vi "ReadABLEConfiguration.vi"(8 "Error In":errorcluster, 11 "VI Path":path) -> (0 "Error Out":errorcluster, 3 "ABLE Configuration":T1)   [LabVIEW 2012]
uses:
  ABLEConfiguration.ctl
  DisplayConfiguration.ctl
  FolderConfiguration.ctl
  AlarmsConfiguration.ctl
  Keithley6485Configuration.ctl
  Keithley6482Configuration.ctl
  <vilib>/Utility/config.llb/Read Key (Boolean).vi
  <vilib>/Utility/config.llb/NI_LVConfig.lvlib
  libs/LV-Utilities/LV-Utilities.lvlib
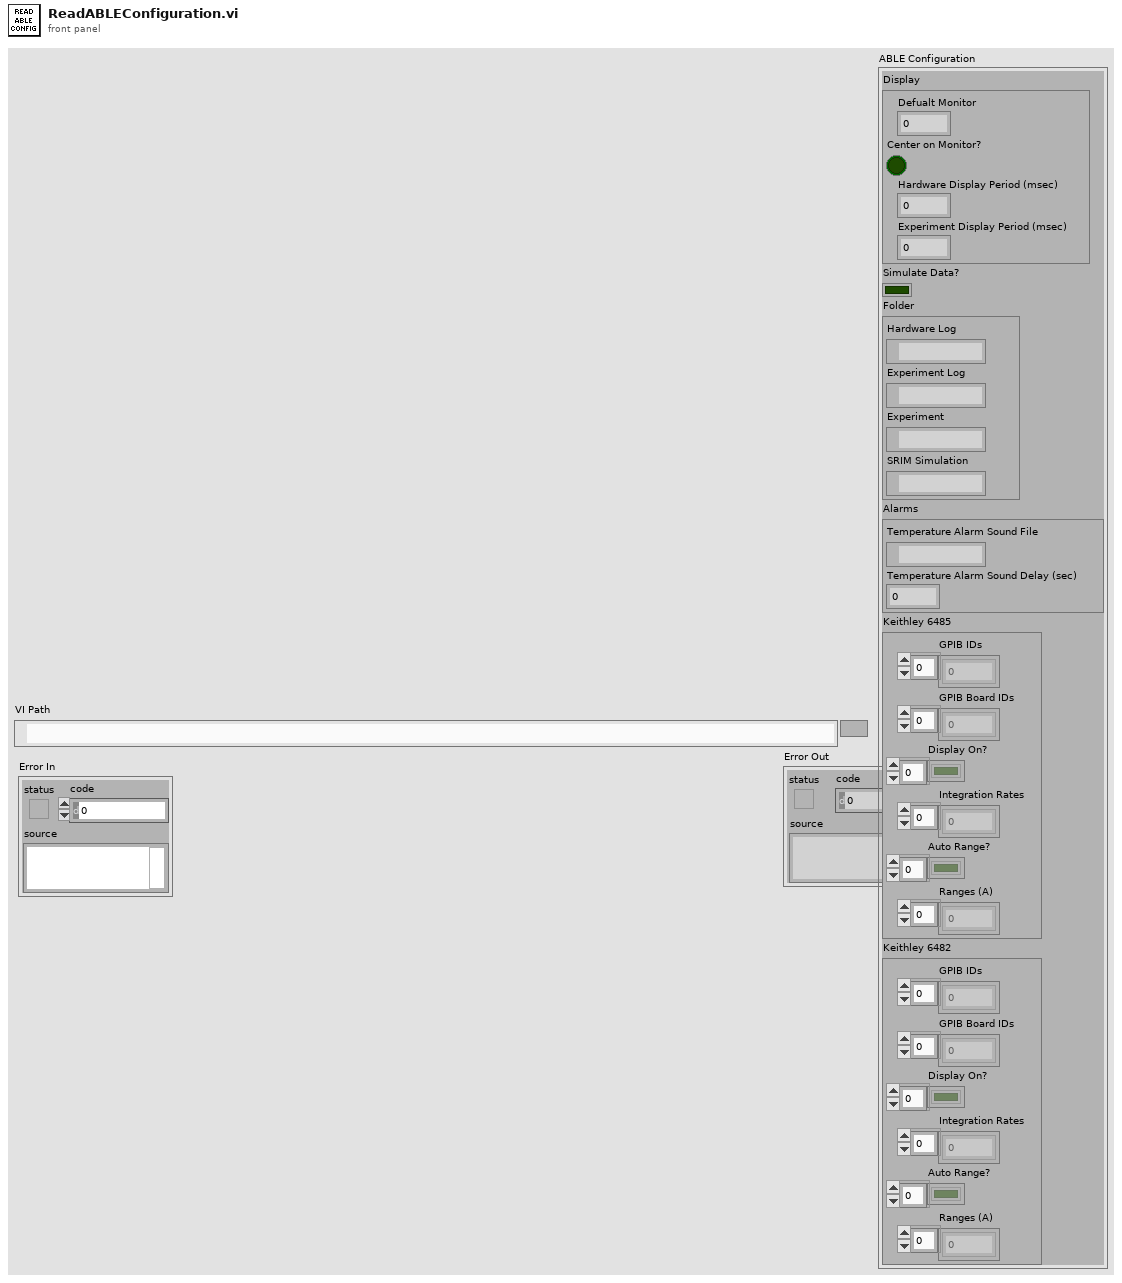
[diagram p1: front panel]
types:
  T1 = typedef "ABLEConfiguration.ctl" = cluster{"Display":T2, "Simulate Data?":bool, "Folder":T3, "Alarms":T4, "Keithley 6485":T5, "Keithley 6482":T6}
  T2 = typedef "DisplayConfiguration.ctl" = cluster{"Defualt Monitor":u16, "Center on Monitor?":bool, "Hardware Display Period (msec)":u32, "Experiment Display Period (msec)":u32}
  T3 = typedef "FolderConfiguration.ctl" = cluster{"Hardware Log":path, "Experiment Log":path, "Experiment":path, "SRIM Simulation":path}
  T4 = typedef "AlarmsConfiguration.ctl" = cluster{"Temperature Alarm Sound File":path, "Temperature Alarm Sound Delay (sec)":dbl}
  T5 = typedef "Keithley6485Configuration.ctl" = cluster{"GPIB IDs":u8[], "GPIB Board IDs":u8[], "Display On?":bool[], "Integration Rates":dbl[], "Auto Range?":bool[], "Ranges (A)":dbl[]}
  T6 = typedef "Keithley6482Configuration.ctl" = cluster{"GPIB IDs":u8[], "GPIB Board IDs":u8[], "Display On?":bool[], "Integration Rates":dbl[], "Auto Range?":bool[], "Ranges (A)":dbl[]}
  T7 = typedef "NI_LVConfig.lvlib/Config Data RefNum.ctl" = refnum<k1>
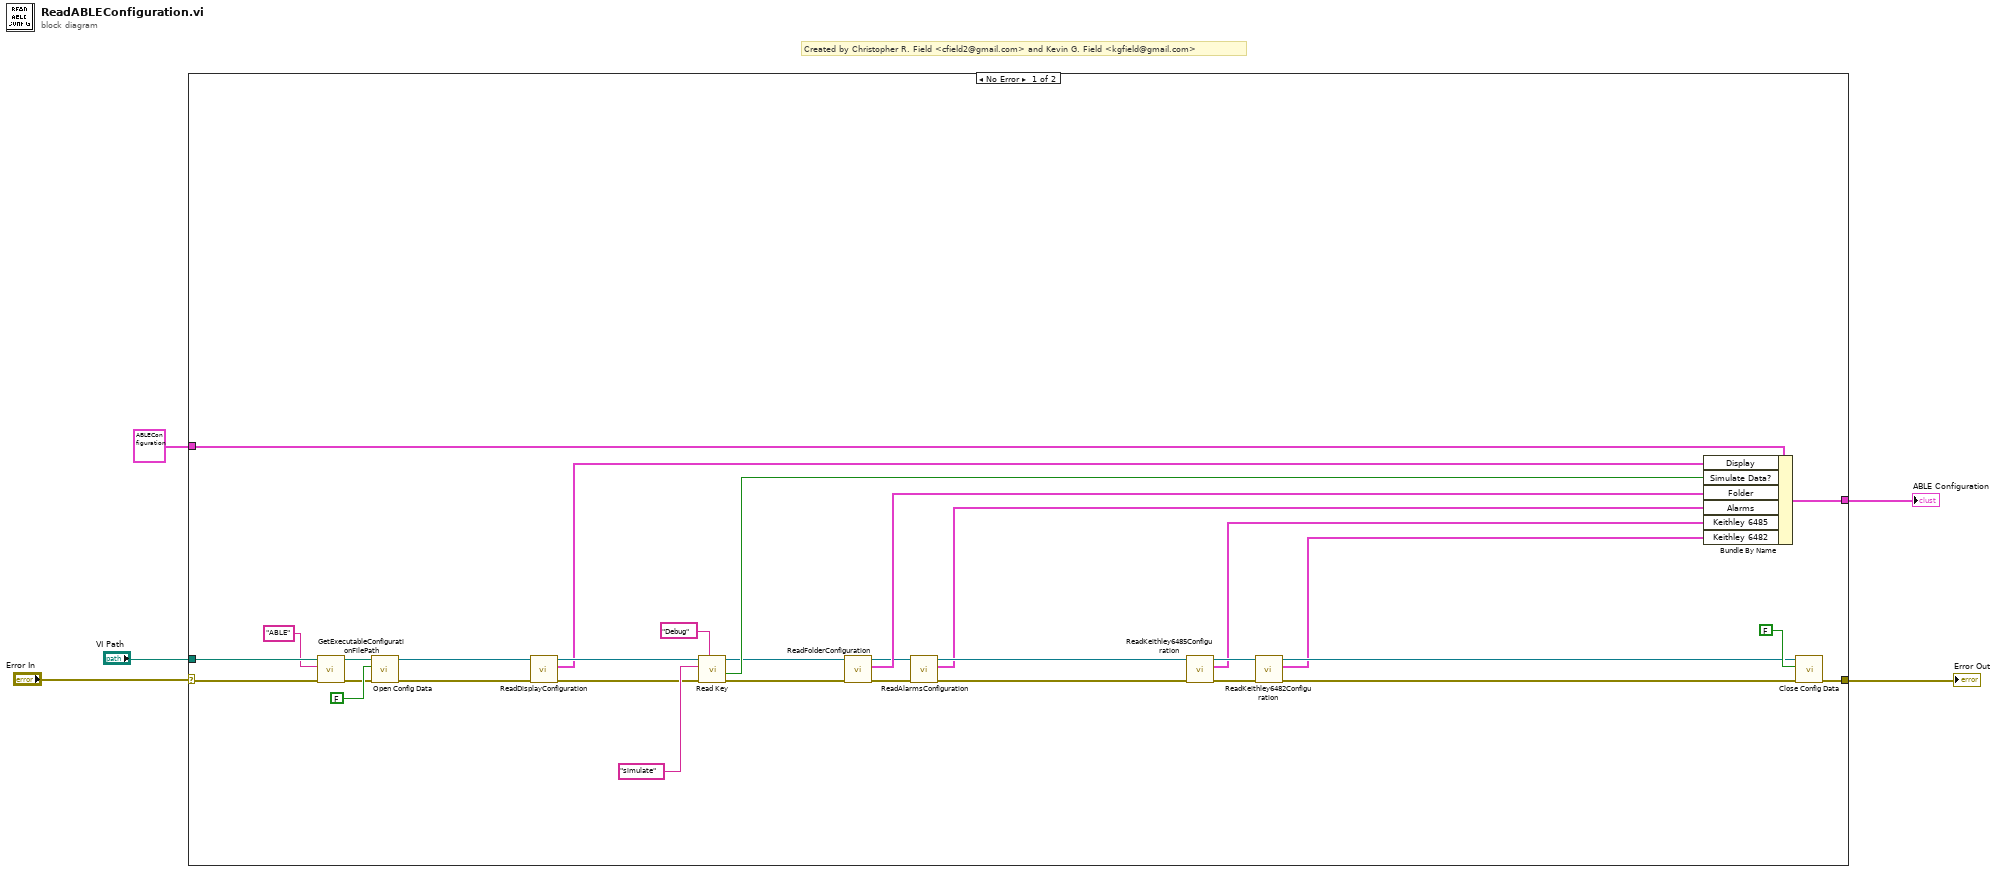
[diagram p0: block diagram]
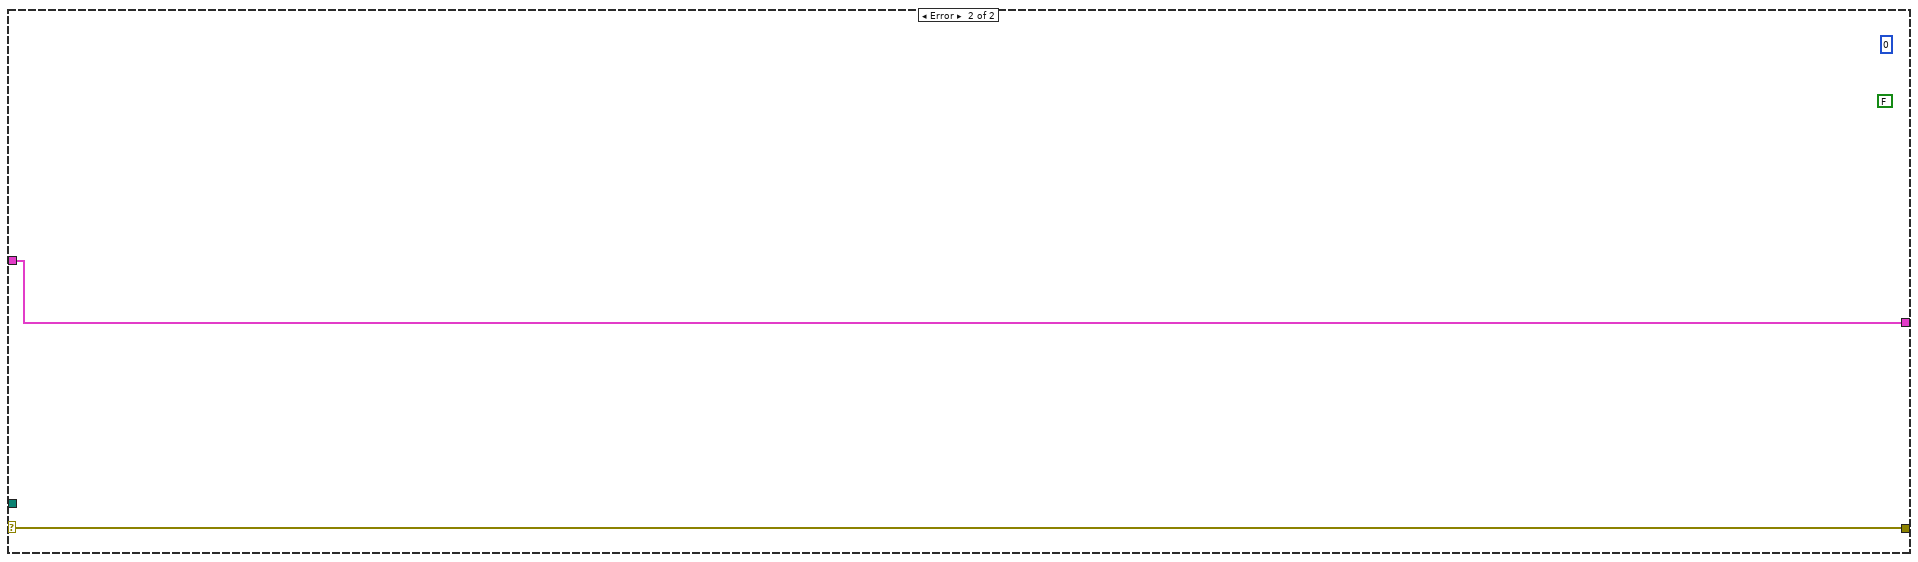
[diagram p2: hidden frame]
diagram:
  # "Created by Christopher R. Field <cfield2@gmail.com> and Kevin G. Field <kgfield@gmail.com>"
  n1 = case shown="No Error" "Error In" {
    selector: "Error In" -> [w14 w39]
    tunnel: "VI Path" -> [w15 _]
    tunnel: [w36 w39] -> w4
    tunnel: [w31 w38] -> w2
    tunnel: T1 {"Display"={"Defualt Monitor"=0, "Center on Monitor?"=FALSE, "Hardware Display Period (msec)"=0, "Experiment Display Period (msec)"=0}, "Simulate Data?"=FALSE, "Folder"={"Hardware Log"=path "", "Experiment Log"=path "", "Experiment"=path "", "SRIM Simulation"=path ""}, "Alarms"={"Temperature Alarm Sound File"=path "", "Temperature Alarm Sound Delay (sec)"=0.0}, "Keithley 6485"={"GPIB IDs"=[], "GPIB Board IDs"=[], "Display On?"=[], "Integration Rates"=[], "Auto Range?"=[], "Ranges (A)"=[]}, "Keithley 6482"={"GPIB IDs"=[], "GPIB Board IDs"=[], "Display On?"=[], "Integration Rates"=[], "Auto Range?"=[], "Ranges (A)"=[]}} ("ABLE Configuration") -> [w30 w38]
    frame No Error {
      n2 = call "GetExecutableConfigurationFilePath.vi"("Error In"=w14, "Application Name"="ABLE", "VI Path"=w15) -> ("Error Out"=w12:errorcluster, "Executable Config File Path"=w13:path)  [unwired: 7 in]
      n3 = call <vilib>:"Open Config Data.vi"("error in (no error)"=w12, "create file if necessary (T)"=FALSE, "configuration file path"=w13) -> ("error out"=w7:errorcluster, "refnum"=w10:T7)  [unwired: 6 in, 1 out]
      n4 = call "ReadDisplayConfiguration.vi"("Error In"=w7, "ABLE Config File Ref In"=w10) -> ("Error Out"=w8:errorcluster, "Display Configuration"=w6:T2, "ABLE Config File Ref Out"=w9:T7)  [unwired: 7 in]
      n5 = call-poly <vilib>:"Read Key.vi"("section"="Debug", "error in (no error)"=w8, "key"="simulate", "refnum"=w9) -> ("error out"=w22:errorcluster, "value"=w32:bool, "refnum out"=w23:T7)  [unwired: 4 in, 1 out]
      n6 = call "ReadFolderConfiguration.vi"("Error In"=w22, "ABLE Config File Ref In"=w23) -> ("Error Out"=w17:errorcluster, "Folder Configuration"=w21:T3, "ABLE Config File Ref Out"=w20:T7)  [unwired: 7 in]
      n7 = call "ReadAlarmsConfiguration.vi"("Error In"=w17, "ABLE Config File Ref In"=w20) -> ("Error Out"=w18:errorcluster, "Alarms Configuration"=w16:T4, "ABLE Config File Ref Out"=w19:T7)  [unwired: 7 in]
      n8 = call "ReadKeithley6485Configuration.vi"("Error In"=w18, "ABLE Config File Ref In"=w19) -> ("Error Out"=w28:errorcluster, "Keithley 6485 Configuration"=w25:T5, "ABLE Config File Ref Out"=w29:T7)  [unwired: 7 in]
      n9 = call "ReadKeithley6482Configuration.vi"("Error In"=w28, "ABLE Config File Ref In"=w29) -> ("Error Out"=w27:errorcluster, "Keithley 6482 Configuration"=w24:T6, "ABLE Config File Ref Out"=w26:T7)  [unwired: 7 in]
      n10 = Bundle By Name(cluster=w30, "Display"=w6, "Simulate Data?"=w32, "Folder"=w21, "Alarms"=w16, "Keithley 6485"=w25, "Keithley 6482"=w24) -> (w31:T1)
      n11 = call <vilib>:"Close Config Data.vi"("error in (no error)"=w27, "write file if changed (T)"=FALSE, "refnum"=w26) -> ("error out"=w36:errorcluster)  [unwired: 7 in, 1 out]
    }
    frame Error {
      (unwired) FALSE ("value")
      (unwired) 0 ("value")
    }
  }
  "Error Out" <- w4
  "ABLE Configuration" <- w2
